vi "MT Demodulate PSK.vi"(0 "input complex waveform":T4={"t0"=0.0, "dt"=1.0, "Y"=[]} {"Y" format="%.3f"; "dt" format="%^.2e"; "t0" format="%.4f"}, 5 "PSK system parameters":T3={"samples per symbol (16)"=16, "symbol map"=[], "differential PSK"=enum."disable", "PSK type"=0} {"PSK type" items=["normal", "shifted", "offset"]; "symbol map" format="%.3f"}, 7 "matched filter coefficients":dbl[](array[numeric]) format="%.2f", 9 "synchronization parameters":T2 {"sync sequence" format="%.2f"}, 11 "error in (no error)":errorcluster, 12 "pulse shaping filter coefficients":dbl[](array[numeric]) format="%.2f", 13 "reset? (T)":bool=TRUE) -> (4 "recovered complex waveform":T4 {"Y" format="%.3f"; "dt" format="%^.2e"; "t0" format="%.4f"}, 6 "output bit stream":i8[](array[numeric]), 8 "measurements":T1 {"phase offset (deg)" format="%.2f"; "frequency drift (Hz)" format="%.2f"; "frequency offset (Hz)" format="%.2f"}, 10 "sync found index (symbols)":dbl format="%.4f", 15 "error out":errorcluster)   [LabVIEW 2020, in "niDMT.lvlib"]
doc: "Demodulates a phase-shift keying (PSK) modulated complex baseband waveform and returns the time-aligned oversampled complex waveform, the demodulated bit stream, and measurement results obtained during demodulation. This VI attempts to remove carrier and phase offset by locking to the carrier signal."
uses:
  <vilib>/addons/Modulation/niDMT.lvlib
  <vilib>/addons/Modulation/Analog/controls/Complex Data Waveform.ctl
  <vilib>/addons/Modulation/Digital/Support/Common/mod_Apply Frequency Offset (Internal).vi
  <vilib>/addons/Modulation/Analog/MT Resample (Complex Cluster).vi
  <vilib>/addons/Modulation/Analog/support/Validators/mod_Fractional Resample Validate.vi
  <vilib>/addons/Modulation/Analog/support/Validators/mod_Check Flush State.vi
  <vilib>/addons/Modulation/Analog/support/mod_FractionalResampler.vi
  <vilib>/addons/Modulation/Analog/support/mod_Integer Rate Interpolation.vi
  <vilib>/addons/Modulation/Analog/support/Validators/mod_Validate Complex Waveform.vi
  <vilib>/addons/Modulation/Analog/support/mod_PerformResampling.vi
  <vilib>/addons/Modulation/Analog/support/Validators/mod_WFErrorHandler.vi
  <vilib>/addons/Modulation/Digital/Support/Common/mod_Truncate FIR Filter (complex).vi
  <vilib>/Utility/error.llb/Error Cluster From Error Code.vi
  <vilib>/addons/Modulation/Analog/support/mod_Resampling Factors.vi
  <vilib>/addons/Modulation/Analog/support/mod_ResamplingFilter.vi
  <vilib>/addons/Modulation/Analog/support/mod_Generate Integer Interpolation Filter.vi
  <vilib>/addons/Modulation/niAMT.lvlib
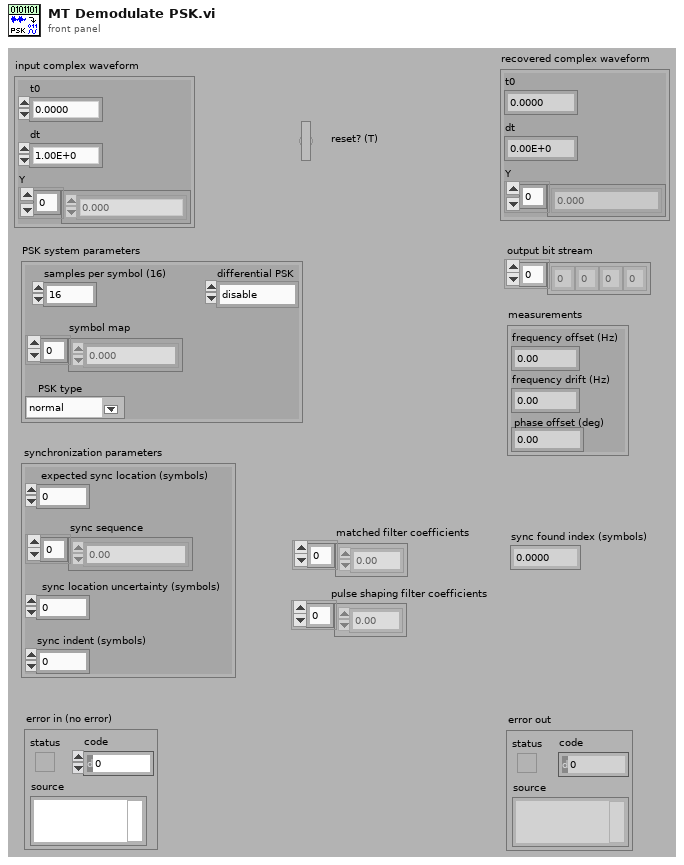
[diagram p1: front panel]
types:
  T1 = cluster{"frequency offset (Hz)":dbl, "frequency drift (Hz)":dbl, "phase offset (deg)":dbl}
  T2 = cluster{"expected sync location (symbols)":i32, "sync sequence":cdb[], "sync location uncertainty (symbols)":i32, "sync indent (symbols)":i32}
  T3 = cluster{"samples per symbol (16)":i32, "symbol map":cdb[], "differential PSK":enum16{"disable", "enable"}, "PSK type":u16}
  T4 = typedef "niAMT.lvlib/Complex Data Waveform.ctl" = cluster{"t0":dbl, "dt":dbl, "Y":cdb[]}
  T5 = enum16{"FSK", "PSK", "QAM", "MSK", "PAM", "ASK", "CPM"}
  T6 = cluster{dbl, "Frequency Drift, Hz":dbl, "Phase Error Estimate, rads":dbl}
  T7 = cluster{"samples per symbol (16)":i32, "symbol map":cdb[], "differential PSK":enum16{"disable", "enable"}}
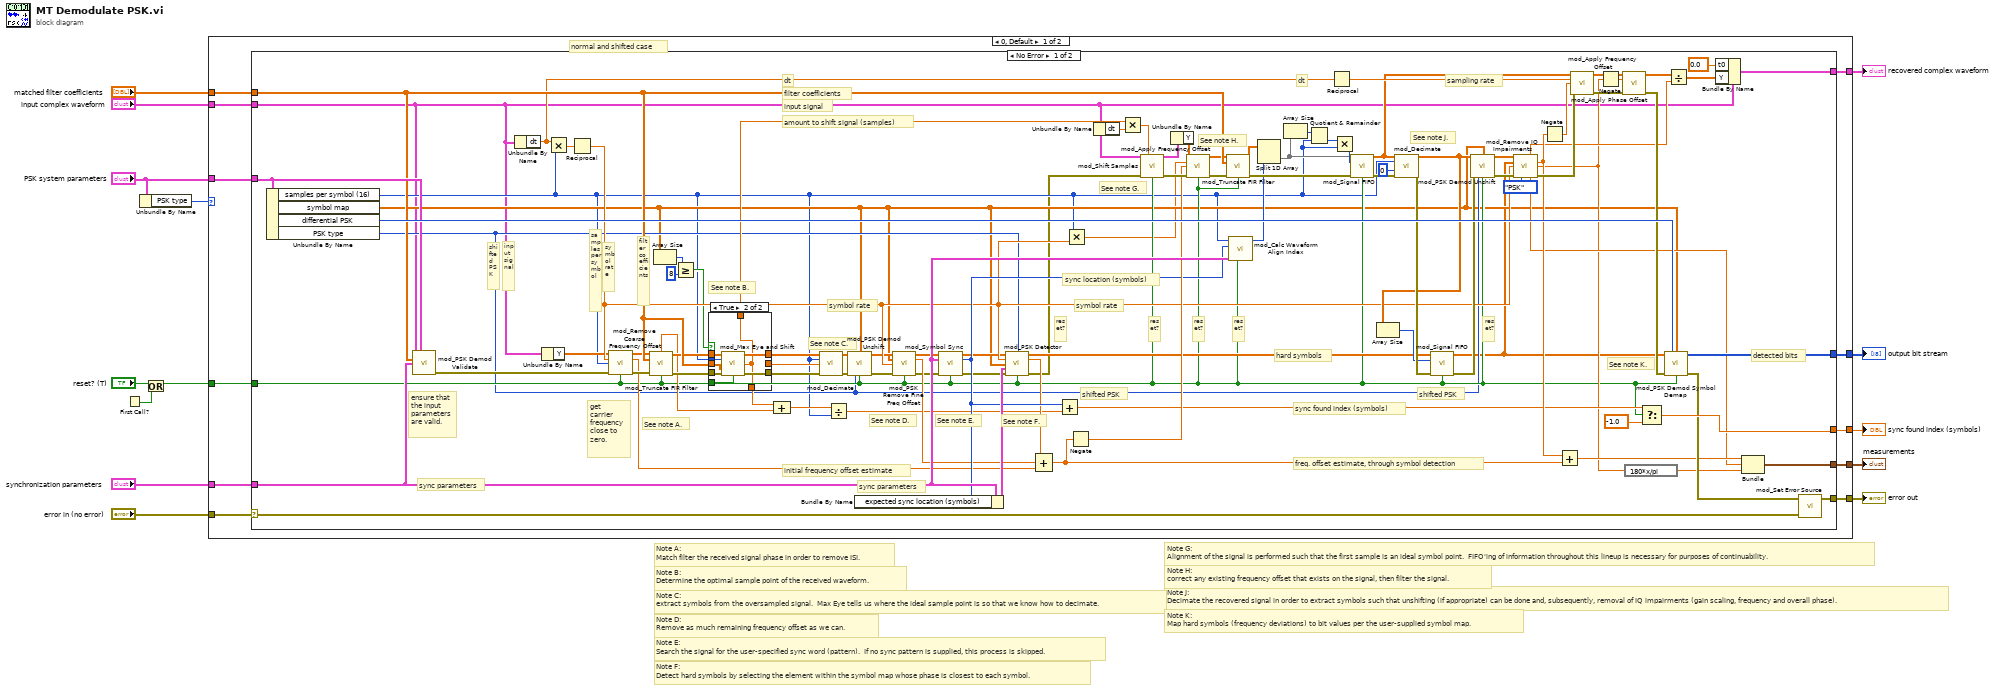
[diagram p0: block diagram]
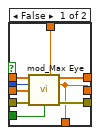
[diagram p2: hidden frame]
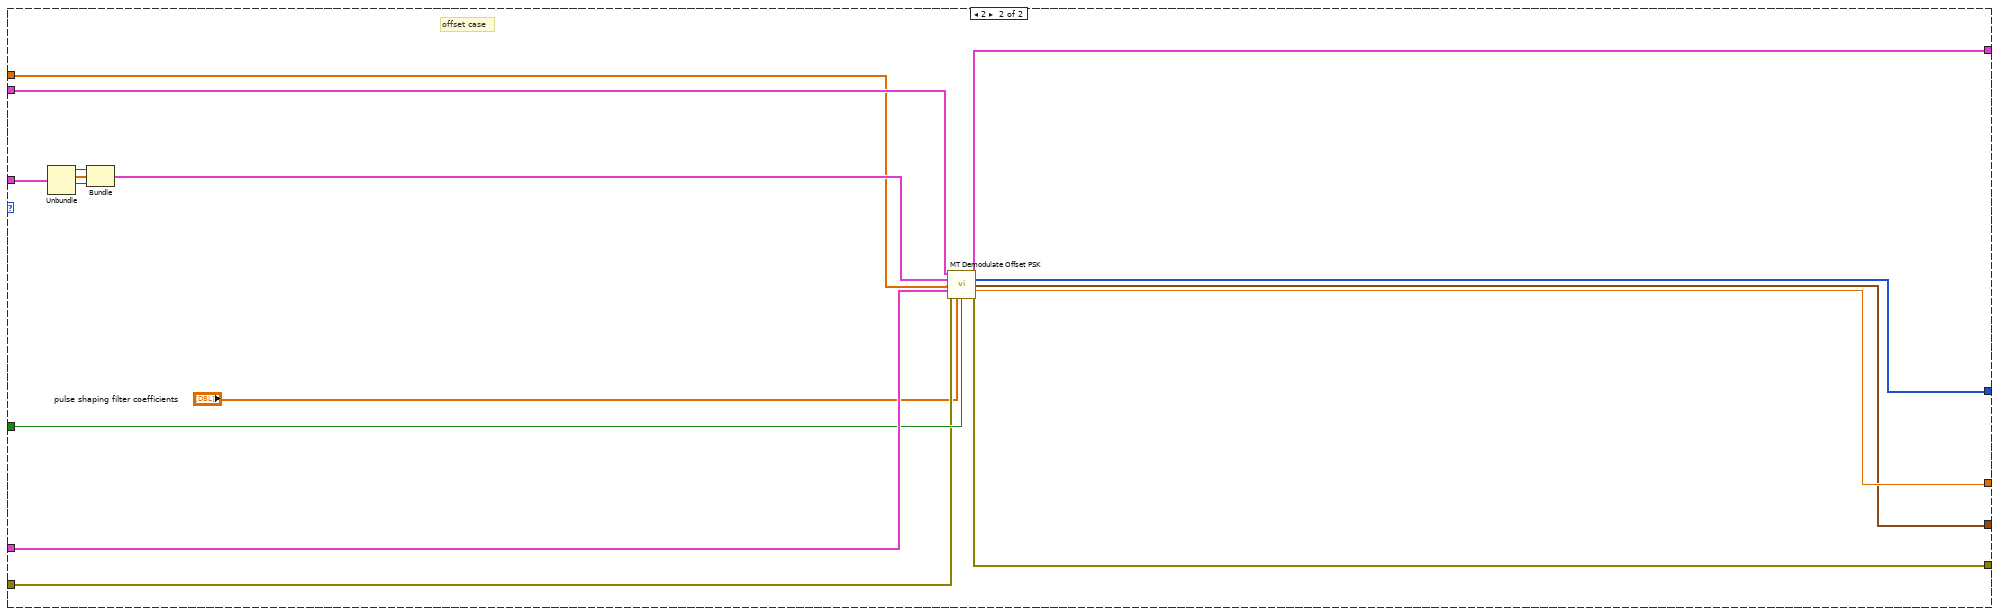
[diagram p4: hidden frame]
diagram:
  # "Note J:\nDecimate the recovered signal in order to extract symbols such that unshifting (if appropriate) can be done and, subsequently, removal of IQ impairments (gain scaling, frequency and overall phase)."
  # "Note H:\ncorrect any existing frequency offset that exists on the signal, then filter the signal."
  # "Note F:\nDetect hard symbols by selecting the element within the symbol map whose phase is closest to each symbol."
  # "Note A:\nMatch filter the received signal phase in order to remove ISI."
  # "Note B:\nDetermine the optimal sample point of the received waveform."
  # "Note C:\nextract symbols from the oversampled signal.  Max Eye tells us where the ideal sample point is so that we know how to decimate."
  # "Note D:\nRemove as much remaining frequency offset as we can."
  # "Note E:\nSearch the signal for the user-specified sync word (pattern).  If no sync pattern is supplied, this process is skipped."
  # "Note G:\nAlignment of the signal is performed such that the first sample is an ideal symbol point.  FIFO'ing of information throughout this lineup is necessary for purposes of continuability."
  # "Note K:\nMap hard symbols (frequency deviations) to bit values per the user-supplied symbol map."
  n1 = First Call?() -> (First Call?: T/F=w5:bool)
  n2 = Unbundle By Name("PSK system parameters") -> ("PSK type"=w1:u16)
  n3 = Or(x="reset? (T)", y=w5) -> (x .or. y?=w3:bool)
  n4 = case shown="0, Default" w1 {
    tunnel: "error in (no error)" -> [w25 w147]
    tunnel: "input complex waveform" -> [w24 w151]
    tunnel: [w23 w141] -> w12
    tunnel: "matched filter coefficients" -> [w22 w150]
    tunnel: [w21 w143] -> w10
    tunnel: "synchronization parameters" -> [w20 w149]
    tunnel: [w19 w144] -> w8
    tunnel: [w18 w142] -> w7
    tunnel: [w17 w145] -> w6
    tunnel: w3 -> [w16 w148]
    tunnel: "PSK system parameters" -> [w15 w156]
    frame 0, Default {
      # "normal and shifted case"
      n5 = case shown="No Error" w25 {
        selector: w25 -> [w111 w140]
        tunnel: w16 -> [w39 _]
        tunnel: w24 -> [w27 _]
        tunnel: [w112 w140] -> w23
        tunnel: w22 -> [w115 _]
        tunnel: [w122 _] -> w19
        tunnel: [w118 _] -> w21
        tunnel: [w119 _] -> w17
        tunnel: w15 -> [w116 _]
        tunnel: w20 -> [w114 _]
        tunnel: [w120 _] -> w18
        frame No Error {
          # "get\ncarrier\nfrequency\nclose to\nzero."
          # "sampling rate"
          # "ensure that the input parameters are valid."
          # "symbol rate"
          # "freq. offset estimate, through symbol detection"
          # "sync found index (symbols)"
          # "dt"
          # "dt"
          # "detected bits"
          # "hard symbols"
          # "shifted PSK"
          # "shifted PSK"
          # "reset?"
          # "reset?"
          # "reset?"
          # "reset?"
          # "reset?"
          # "sync location (symbols)"
          # "symbol rate"
          # "filter coefficients"
          # "amount to shift signal (samples)"
          # "input signal"
          # "initial frequency offset estimate"
          # "sync parameters"
          # "sync parameters"
          # "filter coefficients"
          # "samples per symbol"
          # "input signal"
          # "shifted PSK"
          # "See note A."
          # "See note B."
          # "ensure that\nthe input\nparameters\nare valid."
          # "See note C."
          # "See note D."
          # "See note E."
          # "See note F."
          # "See note G."
          # "See note H."
          # "See note J."
          # "See note K."
          # "symbol rate"
          n6 = Unbundle By Name(w116) -> ("samples per symbol (16)"=w31:i32, "symbol map"=w35:cdb[], "differential PSK"=w121:enum16{"disable", "enable"}, "PSK type"=w37:u16)
          n7 = call <vilib>:"mod_PSK Demod Validate.vi"("Input Complex Waveform"=w27, "PSK System Parameters"=w116, "Matched Filter Coefficients"=w115, "Synchronization Parameters"=w114) -> ("error out"=w117:errorcluster)  [unwired: 3 in, 8 out]
          n8 = Unbundle By Name(w27) -> ("dt"=w89:dbl)
          n9 = Unbundle By Name(w27) -> ("Y"=w49:cdb[])
          n10 = Multiply(x=w89, y=w31) -> (x*y=w90:dbl)
          n11 = Reciprocal(x=w90) -> (1/x=w62:dbl)
          n12 = call <vilib>:"mod_Remove Coarse Frequency Offset.vi"("Signal In"=w49, "Symbol Rate, Hz"=w62, "Samples Per Symbol (16)"=w31, "error in (no error)"=w117, "Reset? (T)"=w39) -> ("Signal Out"=w48:cdb[], "Freq Est, Hz"=w58:dbl, "error out"=w109:errorcluster)  [unwired: 3 in, 5 out]
          n13 = call-poly <vilib>:"mod_Truncate FIR Filter.vi"("Signal In"=w48, "Filter Coefficients"=w115, "error in (no error)"=w109, "Reset? (T)"=w39) -> ("Fractional Delay (samples)"=w46:dbl, "Signal Out"=w84:cdb[], "error out"=w83:errorcluster)  [unwired: 8 in, 1 out]
          n14 = Array Size(array=w35) -> (size(s)=w34:i32)
          n15 = Greater Or Equal?(x=w34, y=8) -> (x >= y?=w32:bool)
          n16 = case shown="True" w32 {
            tunnel: w31 -> [w131 w133]
            tunnel: w115 -> [w130 w132]
            tunnel: w84 -> [w129 w139]
            tunnel: w83 -> [w128 w138]
            tunnel: [w127 w134] -> w45
            tunnel: [w123 w134] -> w44
            tunnel: [w126 w135] -> w43
            tunnel: [w125 w136] -> w42
            tunnel: w39 -> [w124 w137]
            tunnel: [w123 _] -> w36
            frame False {
              n17 = call <vilib>:"mod_Max Eye.vi"("Signal In"=w129, "Samples Per Symbol (16)"=w131, "Filter Coefficients"=w130, "error in (no error)"=w128, "Reset? (T)"=w124) -> ("Waveform Alignment Offset"=w127:dbl, "Signal Out"=w126:cdb[], "Optimal Offset (samples)"=w123:dbl, "error out"=w125:errorcluster)  [unwired: 1 in, 6 out]
            }
            frame True {
              n18 = call <vilib>:"mod_Max Eye and Shift.vi"("Signal In"=w139, "Samples Per Symbol (16)"=w133, "matched filter coefficients"=w132, "error in (no error)"=w138, "Reset? (T)"=w137) -> ("Signal Out"=w135:cdb[], "Optimal Offset (in Samples)"=w134:dbl, "error out"=w136:errorcluster)  [unwired: 8 in]
            }
          }
          n19 = Compound Arithmetic op=ADD(w44, w46) -> (w47:dbl)
          n20 = call <vilib>:"mod_Decimate.vi"("Signal In"=w43, "Samples Per Symbol (16)"=w31, "Offset"=w36, "error in (no error)"=w42) -> ("Signal Out"=w52:cdb[], "error out"=w100:errorcluster)  [unwired: 10 out]
          n21 = Divide(x=w47, y=w31) -> (x/y=w30:dbl)
          n22 = call <vilib>:"mod_PSK Demod Unshift.vi"("Signal In"=w52, "Symbol Map"=w35, "error in (no error)"=w100, "Shifted PSK Enable (disable)"=w37, "Reset? (T)"=w39) -> ("Unshifted Signal"=w51:cdb[], "error out"=w57:errorcluster)  [unwired: 2 in, 7 out]
          n23 = call <vilib>:"mod_PSK Remove Fine Freq Offset.vi"("Symbols"=w51, "Symbol Map"=w35, "Symbol Rate, Hz"=w62, "error in (no error)"=w57, "Reset? (T)"=w39) -> ("Symbols"=w50:cdb[], "Freq Est, Hz"=w61:dbl, "error out"=w56:errorcluster)  [unwired: 8 out]
          n24 = call <vilib>:"mod_Symbol Sync.vi"("Signal In"=w50, "Synchronization Parameters"=w114, "error in (no error)"=w56, "Reset? (T)"=w39) -> ("Signal Out"=w54:cdb[], "Sync Location (symbols)"=w63:i32, "error out"=w55:errorcluster)  [unwired: 1 in, 8 out]
          n25 = Bundle By Name(cluster=w114, "expected sync location (symbols)"=w63) -> (w103:T2)
          n26 = call <vilib>:"mod_PSK Detector.vi"("Signal In"=w54, "PSK type"=w37, "Symbol Rate, Hz"=w62, "Symbol Map"=w35, "Synchronization Parameters"=w103, "error in (no error)"=w55, "Reset (T)"=w39) -> ("Signal Out"=w74:cdb[], "Freq Est, Hz"=w60:dbl, "error out"=w28:errorcluster)  [unwired: 6 out]
          n27 = Compound Arithmetic op=ADD(w60, w61, w58) -> (w59:dbl)
          n28 = Add(x=w63, y=w30) -> (x+y=w73:dbl)
          n29 = Multiply(x=w31, y=w62) -> (x*y=w26:dbl)
          n30 = Negate(x=w59) -> (-x=w101:dbl)
          n31 = Unbundle By Name(w27) -> ("dt"=w53:dbl)
          n32 = Multiply(x=w45, y=w53) -> (x*y=w104:dbl)
          n33 = call <vilib>:"mod_Shift Samples.vi"("Input Complex Waveform"=w27, "Initial Sample Offset, sec"=w104, "error in (no error)"=w28, "Reset? (T)"=w39) -> ("Output Complex Waveform"=w107:T4, "error out"=w105:errorcluster)  [unwired: 10 in]
          n34 = Unbundle By Name(w107) -> ("Y"=w106:cdb[])
          n35 = call <vilib>:"mod_Apply Frequency Offset.vi"("Signal In"=w106, "Rate, pts/sec"=w26, "Freq Offset, Hz"=w101, "error in (no error)"=w105, "Reset? (T)"=w39) -> ("Signal Out"=w110:cdb[], "error out"=w108:errorcluster)  [unwired: 9 out]
          n36 = call-poly <vilib>:"mod_Truncate FIR Filter.vi"("Signal In"=w110, "Filter Coefficients"=w115, "error in (no error)"=w108, "Reset? (T)"=w39) -> ("Signal Out"=w66:cdb[], "error out"=w82:errorcluster)  [unwired: 8 in, 2 out]
          n37 = call <vilib>:"mod_Calc Waveform Align Index.vi"("Reset? (T)"=w39, "Synchronization Parameters"=w114, "Sync Location, symbols"=w63, "Samples Per Symbol (16)"=w31) -> ("align index, samples"=w65:i32)  [unwired: 7 out]
          n38 = Split 1D Array(array=w66, index=w65) -> (second subarray=w67:cdb[])  [unwired: 1 out]
          n39 = Array Size(array=w67) -> (size(s)=w81:i32)
          n40 = Quotient & Remainder(x=w81, y=w31) -> (floor(x/y)=w80:i32)  [unwired: 1 out]
          n41 = Reciprocal(x=w89) -> (1/x=w88:dbl)
          n42 = Multiply(x=w80, y=w31) -> (x*y=w79:i32)
          n43 = call <vilib>:"mod_Signal FIFO.vi"("Signal In"=w67, "Output Length"=w79, "error in (no error)"=w82, "Reset? (T)"=w39) -> ("Signal Out"=w68:cdb[], "error out"=w78:errorcluster)  [unwired: 10 out]
          n44 = call <vilib>:"mod_Decimate.vi"("Signal In"=w68, "Samples Per Symbol (16)"=w31, "Offset"=0, "error in (no error)"=w78) -> ("Signal Out"=w64:cdb[], "error out"=w77:errorcluster)  [unwired: 1 in, 9 out]
          n45 = Array Size(array=w64) -> (size(s)=w75:i32)
          n46 = call <vilib>:"mod_Signal FIFO.vi"("Signal In"=w74, "Output Length"=w75, "error in (no error)"=w77, "Reset? (T)"=w39) -> ("Signal Out"=w29:cdb[], "error out"=w76:errorcluster)  [unwired: 10 out]
          n47 = call <vilib>:"mod_PSK Demod Unshift.vi"("Signal In"=w64, "Symbol Map"=w35, "error in (no error)"=w76, "Shifted PSK Enable (disable)"=w37, "Reset? (T)"=w39) -> ("Unshifted Signal"=w70:cdb[], "error out"=w99:errorcluster)  [unwired: 2 in, 7 out]
          n48 = call <vilib>:"mod_Remove IQ Impairments.vi"("Received Signal In"=w70, "Reference Signal"=w29, "Signal Rate, Hz"=w62, "error in (no error)"=w99, "Modulation Type"=T5."PSK") -> ("Gain Error Estimate"=w86:dbl, "Frequency Estimate, Hz"=w93:dbl, "Phase Error Estimate, rads"=w69:dbl, "Frequency Drift, Hz"=w85:dbl, "error out"=w96:errorcluster)  [unwired: 6 out]
          n49 = Negate(x=w93) -> (-x=w92:dbl)
          n50 = Add(x=w93, y=w59) -> (x+y=w102:dbl)
          n51 = call <vilib>:"mod_Apply Frequency Offset.vi"("Signal In"=w68, "Rate, pts/sec"=w88, "Freq Offset, Hz"=w92, "error in (no error)"=w96) -> ("Signal Out"=w97:cdb[], "error out"=w95:errorcluster)  [unwired: 1 in, 9 out]
          n52 = Negate(x=w69) -> (-x=w91:dbl)
          n53 = call <vilib>:"mod_Apply Phase Offset.vi"("Signal In"=w97, "Phase Offset, rad (0 rad)"=w91, "error in (no error)"=w95) -> ("Signal Out"=w40:cdb[], "error out"=w94:errorcluster)  [unwired: 11 out]
          n54 = expression code="180*x/pi"(w69) -> (w87:dbl)
          n55 = Select(t=w73, s=w39, f=-1.0) -> (s? t:f=w118:dbl)
          n56 = call <vilib>:"mod_PSK Demod Symbol Demap.vi"("Symbols In"=w29, "Differential PSK Enable"=w121, "Symbol Map"=w35, "error in (no error)"=w94, "Reset? (T)"=w39) -> ("Bits Out"=w122:i8[], "error out"=w113:errorcluster)  [unwired: 1 in, 8 out]
          n57 = Divide(x=w40, y=w86) -> (x/y=w71:cdb[])
          n58 = Bundle By Name(cluster=w27, "t0"=0.0, "Y"=w71) -> (w119:T4)
          n59 = Bundle(w102, "Frequency Drift, Hz"=w85, "Phase Error Estimate, rads"=w87) -> (w120:T6)  [unwired: 1 out]
          n60 = call <vilib>:"mod_Set Error Source.vi"("initial error in (no error)"=w111, "final error in (no error)"=w113) -> ("error out"=w112:errorcluster)  [unwired: 3 out]
        }
        frame Error {
        }
      }
    }
    frame 2 {
      # "offset case"
      n61 = Unbundle(w156) -> ("samples per symbol (16)"=w155:i32, "symbol map"=w154:cdb[], "differential PSK"=w153:enum16{"disable", "enable"})  [unwired: 1 out]
      n62 = Bundle("samples per symbol (16)"=w155, "symbol map"=w154, "differential PSK"=w153) -> (w152:T7)  [unwired: 1 out]
      n63 = call <vilib>:"MT Demodulate Offset PSK.vi"("input complex waveform"=w151, "Offset PSK system parameters"=w152, "matched filter coefficients"=w150, "synchronization parameters"=w149, "error in (no error)"=w147, "pulse shaping filter coefficients"="pulse shaping filter coefficients", "reset? (T)"=w148) -> ("recovered complex waveform"=w145:T4, "output bit stream"=w144:i8[], "measurements"=w142:T1, "sync found index (symbols)"=w143:dbl, "error out"=w141:errorcluster)  [unwired: 4 in]
    }
  }
  "error out" <- w12
  "sync found index (symbols)" <- w10
  "output bit stream" <- w8
  "recovered complex waveform" <- w6
  "measurements" <- w7
